vi "MotorClickMove.vi"(0 "error in":errorcluster caption="entrée d'erreur", 5 "Motor steps / click":i32(slide)=100 min=100 max=1000 step=100 scale=1.0..1000.0, 6 "Motors":string[](array[string]), 7 "-Axis":bool[](array[boolean]), 8 "+Axis":bool[](array[boolean])) -> (3 "error out":errorcluster caption="sortie d'erreur", 9 "Motors out":string[](array[string]))   [LabVIEW 2009]
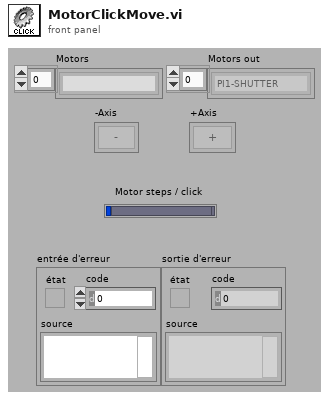
[diagram p1: front panel]
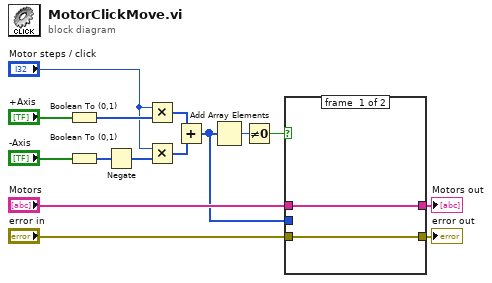
[diagram p0: block diagram]
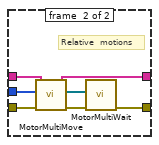
[diagram p2: hidden frame]
diagram:
  n1 = Boolean To (0,1)(Boolean="+Axis") -> (0, 1=w14:i16[])
  n2 = Boolean To (0,1)(Boolean="-Axis") -> (0, 1=w15:i16[])
  n3 = Negate(x=w15) -> (-x=w13:i16[])
  n4 = Multiply(x="Motor steps / click", y=w14) -> (x*y=w11:i32[])
  n5 = Multiply(x="Motor steps / click", y=w13) -> (x*y=w12:i32[])
  n6 = Add(x=w11, y=w12) -> (x+y=w3:i32[])
  n7 = Add Array Elements(numeric array=w3) -> (sum=w2:i32)
  n8 = Not Equal To 0?(x=w2) -> (x != 0?=w1:bool)
  n9 = case shown="True" w1 {
    tunnel: "error in" -> [w16 w24]
    tunnel: "Motors" -> [w17 w23]
    tunnel: [w16 w21] -> w5
    tunnel: [w17 w19] -> w4
    tunnel: w3 -> [_ w18]
    frame #0 {
    }
    frame #1 {
      # "Relative  motions"
      n10 = call "MotorMultiMove.vi"("Motors"=w23, "Positions"=w18, "error in (no error)"=w24) -> ("Motors out"=w19:string[], "Ok?"=w20:refnum<k4>[], "error out"=w22:errorcluster)  [unwired: 4 in]
      n11 = call "MotorMultiWait.vi"("Ok?"=w20, "error out"=w22) -> ("error in (no error)"=w21:errorcluster)  [unwired: 7 in]
    }
  }
  "error out" <- w5
  "Motors out" <- w4
